vi "Configure RAMP DOWN.vi"(7 "All Channels (F)":bool, 8 "error in (no error)":errorcluster, 9 "Voltage ramp down (0 V/s)":u16 max=999, 10 "Channel (0)":u8, 11 "BoardHandle":T1) -> (0 "error out":errorcluster, 3 "BoardHandle out":T1)   [LabVIEW 2018, in "CAEN PSM.lvlib"]
doc: "This function allows to configure Voltage Ramp Down rate."
uses:
  CAEN PSM.lvlib
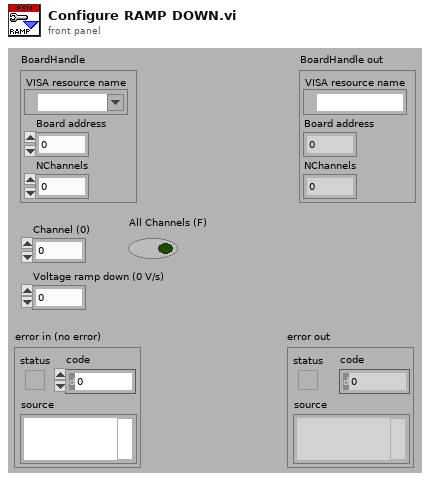
[diagram p1: front panel]
types:
  T1 = cluster{"VISA resource name":refnum<visa-resource-name>, "Board address":u8, "NChannels":u8}
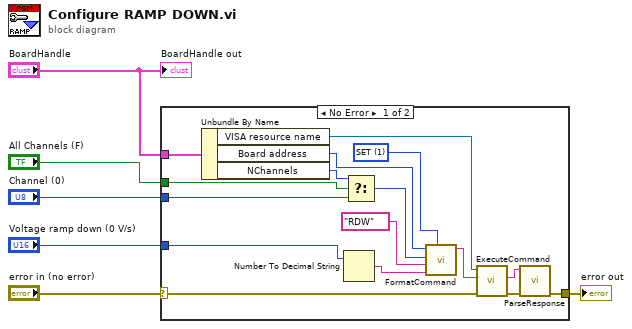
[diagram p0: block diagram]
diagram:
  n1 = case shown="No Error" "error in (no error)" {
    selector: "error in (no error)" -> [w10 w23]
    tunnel: "All Channels (F)" -> [w20 _]
    tunnel: "Channel (0)" -> [w18 _]
    tunnel: [w13 w23] -> w3
    tunnel: "BoardHandle" -> [w11 _]
    tunnel: "Voltage ramp down (0 V/s)" -> [w8 _]
    frame No Error {
      w21 = u8 1 items=["MON", "SET"] ("CMD")
      n2 = Unbundle By Name(w11) -> ("VISA resource name"=w16:refnum<visa-resource-name>, "Board address"=w22:u8, "NChannels"=w19:u8)
      n3 = Number To Decimal String(number=w8) -> (decimal integer string=w7:string)  [unwired: 1 in]
      n4 = Select(t=w19, s=w20, f=w18) -> (s? t:f=w17:u8)
      n5 = call "FormatCommand.vi"("CMD (MON)"=w21, "VAL"=w7, "PAR"="RDW", "CH"=w17, "BD (0)"=w22) -> ("cmd"=w15:string)  [unwired: 6 in]
      n6 = call "ExecuteCommand.vi"("error in (no error)"=w10, "Command"=w15, "VISA resource name"=w16) -> ("error out"=w14:errorcluster, "Response"=w12:string)  [unwired: 6 in, 1 out]
      n7 = call "ParseResponse.vi"("error in (no error)"=w14, "Response"=w12) -> ("error out"=w13:errorcluster)  [unwired: 6 in, 3 out]
    }
    frame Error {
    }
  }
  "error out" <- w3
  "BoardHandle out" <- "BoardHandle"
